vi "excavator2D.vi"() -> ()   [LabVIEW 2013]
panel:
  in  "ampl":dbl[][](graph)=array7x3900[27300 elements]
  in  "Tab Control":enum32{"Page 1", "Page 2"}(tab)
  in  "x Max":dbl=-40.0 format="%#_13g"
  in  "x Min":dbl=-50.0 format="%#_13g"
  in  "y Min":dbl format="%#_13g"
  in  "y Max":dbl=15.0 format="%#_13g"
  in  "?":bool=TRUE
  in  "Limits":bool
  out "xPoints":i32=451
  out "yPoints":i32=851
  in  "matrix?":bool=TRUE
  in  "file path (use dialog)":path
  # "XYZ file \n#no_x by no_y\nx1 y1 z1\nx1 y2 z2\nx1 y3 z3\n...\nx4 y1 z?"
  # "Matrix file\n#xrange\n#yrange\nz11 z12 z13 ...\nz21 z22 z23 ..."
  # "Data on graph"
  # "All Data"
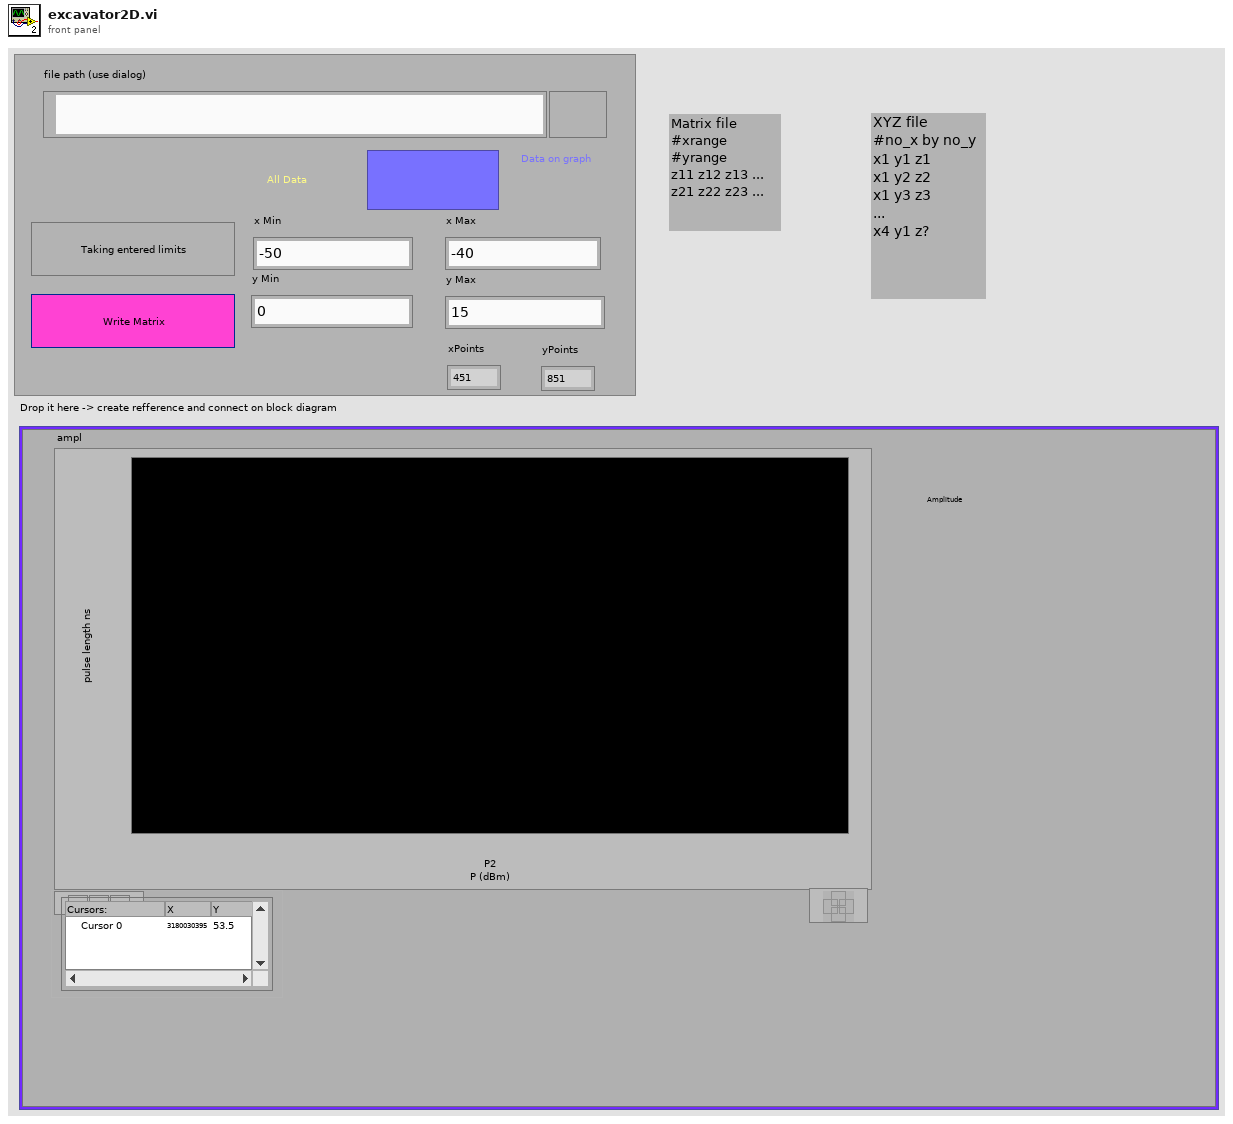
[diagram p1: front panel]
types:
  T1 = enum16{"open", "replace", "create", "open or create", "replace or create", "replace or create with confirmation"}
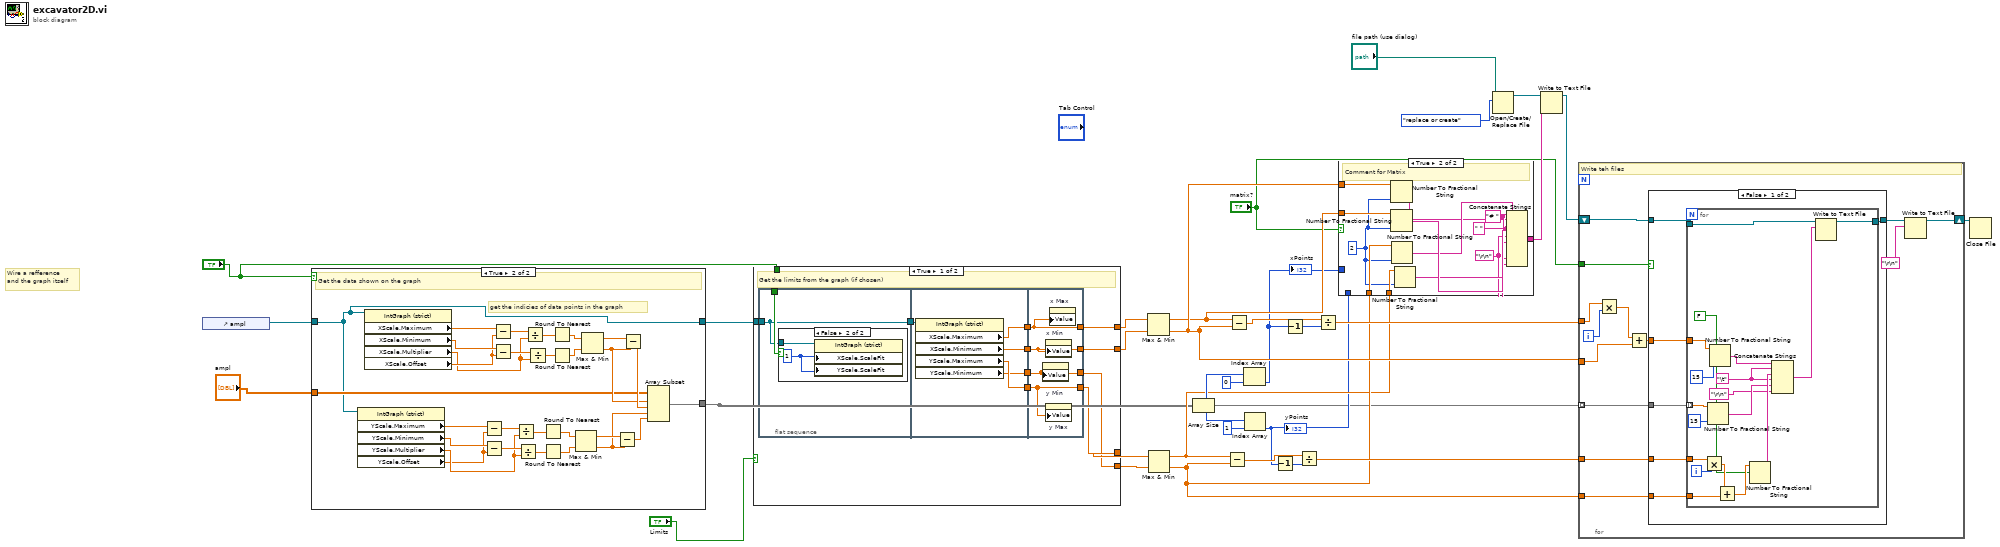
[diagram p0: block diagram]
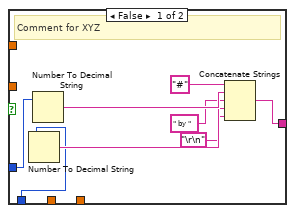
[diagram p2: hidden frame]
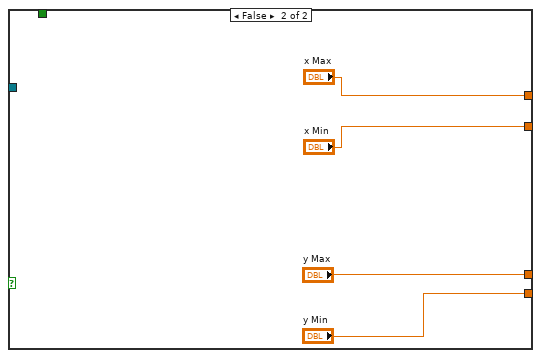
[diagram p5: hidden frame]
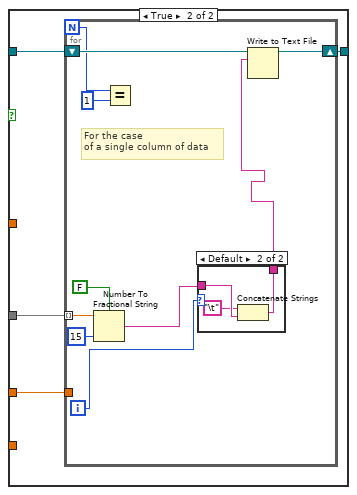
[diagram p6: hidden frame]
diagram:
  # "Wire a refference\nand the graph itself"
  n1 = control-ref of="ampl"() -> (w7:refnum<vi>)
  n2 = case shown="True" "?" {
    tunnel: "ampl" -> [w34 w42]
    tunnel: w7 -> [w33 w35]
    tunnel: [w34 w36] -> w3
    tunnel: [w33 w35] -> w24
    frame False {
    }
    frame True {
      # "get the indicies of data points in the graph"
      # "Get the data shown on the graph"
      n3 = property class="IntGraph (strict)"(reference=w35) -> ("YScale.Maximum"=w51:dbl, "YScale.Minimum"=w50:dbl, "YScale.Multiplier"=w49:dbl, "YScale.Offset"=w48:dbl)  [unwired: 1 in, 2 out]
      n4 = property class="IntGraph (strict)"(reference=w35) -> ("XScale.Maximum"=w60:dbl, "XScale.Minimum"=w63:dbl, "XScale.Multiplier"=w56:dbl, "XScale.Offset"=w57:dbl)  [unwired: 1 in, 2 out]
      n5 = Subtract(x=w51, y=w48) -> (x-y=w53:dbl)
      n6 = Subtract(x=w50, y=w48) -> (x-y=w52:dbl)
      n7 = Subtract(x=w60, y=w57) -> (x-y=w61:dbl)
      n8 = Subtract(x=w63, y=w57) -> (x-y=w62:dbl)
      n9 = Divide(x=w53, y=w49) -> (x/y=w54:dbl)
      n10 = Divide(x=w52, y=w49) -> (x/y=w55:dbl)
      n11 = Divide(x=w61, y=w56) -> (x/y=w59:dbl)
      n12 = Divide(x=w62, y=w56) -> (x/y=w58:dbl)
      n13 = Round To Nearest(number=w54) -> (nearest integer value=w40:dbl)
      n14 = Round To Nearest(number=w55) -> (nearest integer value=w39:dbl)
      n15 = Round To Nearest(number=w59) -> (nearest integer value=w47:dbl)
      n16 = Round To Nearest(number=w58) -> (nearest integer value=w46:dbl)
      n17 = Max & Min(x=w40, y=w39) -> (max(x,y)=w41:dbl, min(x,y)=w37:dbl)
      n18 = Max & Min(x=w47, y=w46) -> (max(x,y)=w44:dbl, min(x,y)=w43:dbl)
      n19 = Subtract(x=w41, y=w37) -> (x-y=w38:dbl)
      n20 = Subtract(x=w44, y=w43) -> (x-y=w45:dbl)
      n21 = Array Subset(array=w42, index (row)=w43, length (row)=w45, index (col)=w37, length (col)=w38) -> (w36:dbl[][])
    }
  }
  n22 = case shown="True" "Limits" {
    tunnel: [w73 "x Max"] -> w22
    tunnel: [w72 "x Min"] -> w21
    tunnel: [w71 "y Max"] -> w20
    tunnel: [w70 "y Min"] -> w19
    tunnel: w24 -> [w74 _]
    tunnel: "?" -> [w68 _]
    frame True {
      # "Get the limits from the graph (if chosen)"
      n23 = flat-sequence {
        tunnel: w74 -> [w75]
        tunnel: [w75] -> w69
        tunnel: w68 -> [w76]
        tunnel: w69 -> [w83]
        tunnel: [w82] -> w67
        tunnel: [w81] -> w66
        tunnel: [w80] -> w65
        tunnel: [w79] -> w64
        tunnel: [w86] -> w70
        tunnel: [w87] -> w71
        tunnel: [w84] -> w72
        tunnel: [w85] -> w73
        tunnel: w67 -> [w85]
        tunnel: w66 -> [w84]
        tunnel: w65 -> [w87]
        tunnel: w64 -> [w86]
        frame #0 {
          n24 = case shown="False" w76 {
            tunnel: w75 -> [_ w77]
            frame True {
            }
            frame False {
              w78 = u8 1 ("X Scale.Scale Fit")
              n25 = property class="IntGraph (strict)"(reference=w77, "XScale.ScaleFit"=w78, "YScale.ScaleFit"=w78) -> ()  [unwired: 1 in, 2 out]
            }
          }
        }
        frame #1 {
          n26 = property class="IntGraph (strict)"(reference=w83) -> ("XScale.Maximum"=w82:dbl, "XScale.Minimum"=w81:dbl, "YScale.Maximum"=w80:dbl, "YScale.Minimum"=w79:dbl)  [unwired: 1 in, 2 out]
        }
        frame #2 {
          n27 = property on="y Min" class="DigNum (strict)"("Value"=w86) -> ()  [unwired: 2 in, 2 out]
          n28 = property on="x Min" class="DigNum (strict)"("Value"=w84) -> ()  [unwired: 2 in, 2 out]
          n29 = property on="y Max" class="DigNum (strict)"("Value"=w87) -> ()  [unwired: 2 in, 2 out]
          n30 = property on="x Max" class="DigNum (strict)"("Value"=w85) -> ()  [unwired: 2 in, 2 out]
        }
      }
    }
    frame False {
    }
  }
  n31 = Max & Min(x=w22, y=w21) -> (max(x,y)=w11:dbl, min(x,y)=w12:dbl)
  n32 = Max & Min(x=w20, y=w19) -> (max(x,y)=w9:dbl, min(x,y)=w10:dbl)
  n33 = Array Size(array=w3) -> (size(s)=w25:i32[])
  n34 = Subtract(x=w9, y=w10) -> (x-y=w27:dbl)
  n35 = Subtract(x=w11, y=w12) -> (x-y=w29:dbl)
  n36 = Index Array(array=w25, index=0) -> (element=w5:i32)
  "xPoints" <- w5
  n37 = Index Array(array=w25, index=1) -> (element=w4:i32)
  "yPoints" <- w4
  n38 = Decrement(x=w4) -> (x-1=w17:i32)
  n39 = Decrement(x=w5) -> (x-1=w18:i32)
  n40 = Divide(x=w27, y=w17) -> (x/y=w30:dbl)
  n41 = Divide(x=w29, y=w18) -> (x/y=w31:dbl)
  n42 = case shown="True" "matrix?" {
    tunnel: [w93 w112] -> w16
    tunnel: w12 -> [_ w111]
    tunnel: w11 -> [_ w110]
    tunnel: w10 -> [_ w107]
    tunnel: w9 -> [_ w103]
    tunnel: w5 -> [w95 _]
    tunnel: w4 -> [w94 _]
    frame False {
      # "Comment for XYZ"
      n43 = Number To Decimal String(number=w94) -> (decimal integer string=w97:string)  [unwired: 1 in]
      n44 = Number To Decimal String(number=w95) -> (decimal integer string=w99:string)  [unwired: 1 in]
      n45 = Concatenate Strings("#" ("string"), w99, " by " ("string"), w97, "\r\n") -> (w93:string)
    }
    frame True {
      w101 = i16 2 ("width (-)")
      w105 = " " ("string")
      w102 = "\r\n"
      w108 = "# " ("string")
      # "Comment for Matrix"
      n46 = Number To Fractional String(number=w111, precision (6)=w101) -> (F-format string=w100:string)  [unwired: 2 in]
      n47 = Number To Fractional String(number=w110, precision (6)=w101) -> (F-format string=w109:string)  [unwired: 2 in]
      n48 = Number To Fractional String(number=w107, precision (6)=w101) -> (F-format string=w106:string)  [unwired: 2 in]
      n49 = Number To Fractional String(number=w103, precision (6)=w101) -> (F-format string=w104:string)  [unwired: 2 in]
      n50 = Concatenate Strings(w108, w100, w105, w109, w102, w108, w106, w105, w104, w102) -> (w112:string)
    }
  }
  n51 = Open/Create/Replace File(file path (use dialog)="file path (use dialog)", operation (0:open)=T1."replace or create") -> (refnum out=w15:refnum<file>)  [unwired: 4 in, 2 out]
  n52 = Write to Text File(file (use dialog)=w15, text=w16) -> (refnum out=w14:refnum<file>)  [unwired: 2 in, 2 out]
  n53 = for {
    tunnel: w3 -> [w125] mode=indexing
    tunnel: w31 -> [w118]
    tunnel: w12 -> [w116]
    tunnel: w10 -> [w114]
    tunnel: w30 -> [w123]
    shift-right: [w121] -> w13
    shift-left: w14 -> [w124]
    tunnel: "matrix?" -> [w113]
    i -> [w117]
    # "Write teh files"
    n54 = Multiply(x=w118, y=w117) -> (x*y=w119:dbl)
    n55 = Add(x=w119, y=w116) -> (x+y=w115:dbl)
    n56 = case shown="False" w113 {
      tunnel: w125 -> [w128 w153]
      tunnel: w124 -> [w131 w152]
      tunnel: w123 -> [w127 w151]
      tunnel: [w130 w150] -> w122
      tunnel: w115 -> [w129 _]
      tunnel: w114 -> [w126 _]
      frame False {
        n57 = for {
          tunnel: w131 -> [w149]
          tunnel: [w139] -> w130
          tunnel: w129 -> [w136]
          tunnel: w128 -> [w135] mode=indexing
          tunnel: w127 -> [w134]
          tunnel: w126 -> [w133]
          i -> [w147]
          w132 = FALSE ("use system decimal point (T)")
          w142 = "\t"
          n58 = Multiply(x=w134, y=w147) -> (x*y=w148:dbl)
          n59 = Number To Fractional String(use system decimal point (T)=w132, number=w135, precision (6)=i16 15) -> (F-format string=w143:string)  [unwired: 1 in]
          n60 = Number To Fractional String(use system decimal point (T)=w132, number=w136, precision (6)=i16 15) -> (F-format string=w146:string)  [unwired: 1 in]
          n61 = Add(x=w148, y=w133) -> (x+y=w145:dbl)
          n62 = Number To Fractional String(use system decimal point (T)=w132, number=w145) -> (F-format string=w144:string)  [unwired: 2 in]
          n63 = Concatenate Strings(w146, w142, w144, w142, w143, "\r\n") -> (w140:string)
          n64 = Write to Text File(file (use dialog)=w149, text=w140) -> (refnum out=w139:refnum<file>)  [unwired: 2 in, 2 out]
        }
      }
      frame True {
        n65 = for {
          N -> [w157]
          tunnel: w153 -> [w162] mode=indexing
          tunnel: w151 -> [_]
          shift-right: [w161] -> w150
          shift-left: w152 -> [w163]
          i -> [w159]
          # "For the case\nof a single column of data"
          n66 = Number To Fractional String(use system decimal point (T)=FALSE, number=w162, precision (6)=i16 15) -> (F-format string=w158:string)  [unwired: 1 in]
          n67 = Equal?(x=w157, y=1) -> ()  [unwired: 1 out]
          n68 = case shown="Default" w159 {
            tunnel: w158 -> [w164 w167]
            tunnel: [w164 w166] -> w155
            frame 0 {
            }
            frame Default {
              n69 = Concatenate Strings("\t" ("string"), w167) -> (w166:string)
            }
          }
          n70 = Write to Text File(file (use dialog)=w163, text=w155) -> (refnum out=w161:refnum<file>)  [unwired: 2 in, 2 out]
        }
      }
    }
    n71 = Write to Text File(file (use dialog)=w122, text="\r\n") -> (refnum out=w121:refnum<file>)  [unwired: 2 in, 2 out]
  }
  n72 = Close File(refnum=w13) -> ()  [unwired: 1 in, 2 out]
